vi "checkAlignment.vi"(5 "Ball":refnum<class "Ball.lvclass">, 6 "target gap":dbl[](array[numeric]), 7 "attacking ourselves":bool, 8 "error in (no error)":errorcluster, 9 "AlignError":T1, 10 "Robot":refnum<class "Robot.lvclass">, 11 "KickToSkill in":refnum<class "KickToSkill.lvclass">) -> (0 "error out":errorcluster, 2 "Aligned":bool, 3 "KickToSkill out":refnum<class "KickToSkill.lvclass">)   [LabVIEW 2023, in "KickToSkill.lvclass"]
uses:
  KickToSkill.lvclass
  Robot_class/Robot.lvclass
  Ball_class/Ball.lvclass
  Robot_class/robotKickToStates.ctl
  Robot_class/Robot.lvclass/Robot.ctl
  Object_class/Read position(x,y).vi
  Robot_class/Read robotKickState.vi
  Robot_class/Read orientation.vi
  Utilities_class/Utilities.lvclass
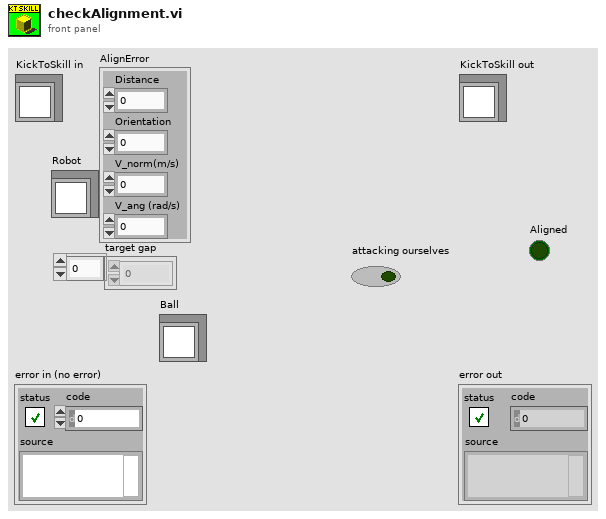
[diagram p1: front panel]
types:
  T1 = cluster{"Distance":dbl, "Orientation":dbl, "V_norm(m/s)":dbl, "V_ang (rad/s)":dbl}
  T2 = typedef "robotKickToStates.ctl" = enum16{"shootFromDirect", "avoidCollideBall", "goToBackBall", "none", "walk", "turn", "turnAntiClockWise", "turnClockwise", "oldKickToShoot", "oldKickToGoToBackBall", "shoot"}
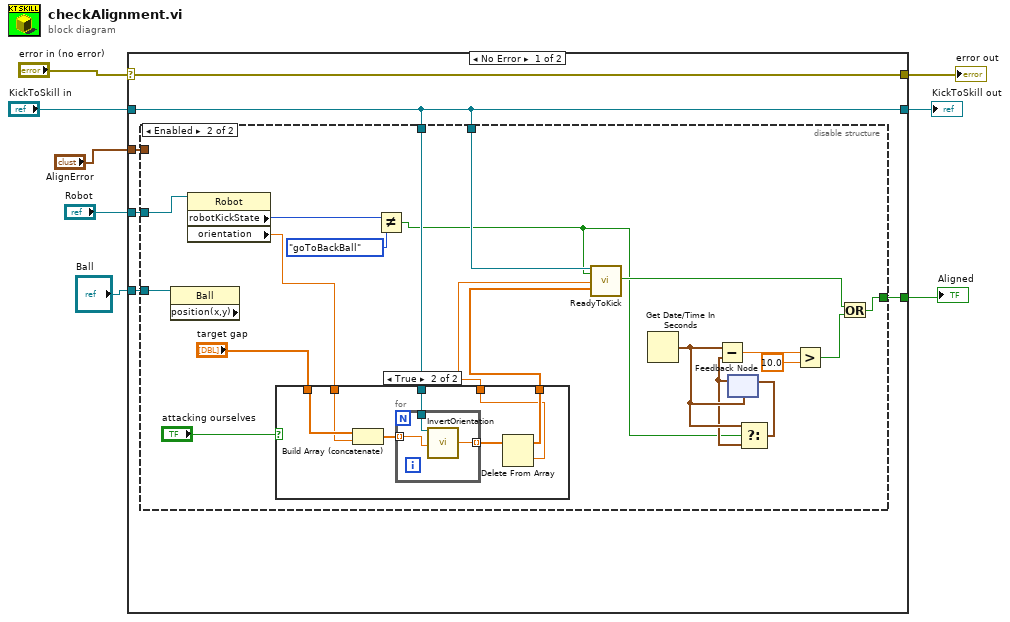
[diagram p0: block diagram]
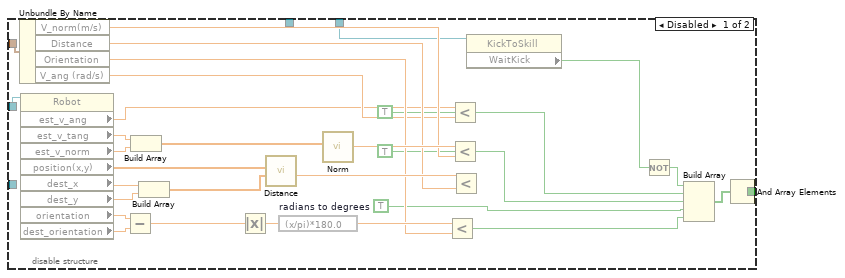
[diagram p2: hidden frame]
diagram:
  n1 = case shown="No Error" "error in (no error)" {
    selector: "error in (no error)" -> [w14 w78]
    tunnel: [w14 w78] -> w7
    tunnel: [w10 w77] -> w5
    tunnel: "KickToSkill in" -> [w10 w77]
    tunnel: "Robot" -> [w13 _]
    tunnel: "AlignError" -> [w12 _]
    tunnel: [w11 _] -> w2
    tunnel: "Ball" -> [w9 _]
    frame No Error {
      n2 = disable-structure shown="Enabled" {
        disable-tunnel: w13 -> [w44 w63]
        disable-tunnel: w12 -> [w29 _]
        disable-tunnel: w10 -> [w23 w64]
        disable-tunnel: [w18 w48] -> w11
        disable-tunnel: w10 -> [_ w57]
        disable-tunnel: w9 -> [_ w56]
        frame Disabled {
          n3 = Unbundle By Name(w29) -> ("V_norm(m/s)"=w28:dbl, "Distance"=w27:dbl, "Orientation"=w26:dbl, "V_ang (rad/s)"=w25:dbl)
          n4 = property class="Robot"(reference=w44) -> ("est_v_ang"=w24:dbl, "est_v_tang"=w32:dbl, "est_v_norm"=w33:dbl, "position(x,y)"=w40:dbl[], "dest_x"=w43:dbl, "dest_y"=w42:dbl, "orientation"=w39:dbl, "dest_orientation"=w38:dbl)  [unwired: 1 in, 2 out]
          n5 = Subtract(x=w39, y=w38) -> (x-y=w37:dbl)
          n6 = Build Array(w32, w33) -> (w31:dbl[])
          n7 = Build Array(w43, w42) -> (w41:dbl[])
          n8 = Absolute Value(x=w37) -> (abs(x)=w36:dbl)
          n9 = call "Distance.vi"("P1"=w41, "P2"=w40) -> ("Distance"=w34:dbl)  [unwired: 7 in, 2 out]
          n10 = expression code="(x/pi)*180.0" "radians to degrees"(w36) -> (w35:dbl)
          n11 = call "Norm.vi"("2D vector"=w31) -> ("Modulo"=w30:dbl)  [unwired: 8 in, 2 out]
          n12 = Less?(x=w35, y=w26) -> (x < y?=w20:bool)
          n13 = Less?(x=w24, y=w25) -> ()  [unwired: 1 out]
          n14 = Less?(x=w30, y=w28) -> ()  [unwired: 1 out]
          n15 = Less?(x=w34, y=w27) -> ()  [unwired: 1 out]
          n16 = property class="KickToSkill"(reference=w23) -> ("WaitKick"=w22:bool)  [unwired: 1 in, 2 out]
          n17 = Not(x=w22) -> (.not. x?=w21:bool)
          n18 = Build Array(w21, TRUE, TRUE, TRUE, w20) -> (w19:bool[])
          n19 = And Array Elements(Boolean array=w19) -> (logical AND=w18:bool)
        }
        frame Enabled {
          n20 = property class="Ball" props=["position(x,y)"](reference=w56) -> ()  [unwired: 1 in, 3 out]
          n21 = property class="Robot"(reference=w63) -> ("robotKickState"=w47:T2, "orientation"=w59:dbl)  [unwired: 1 in, 2 out]
          n22 = case shown="True" "attacking ourselves" {
            tunnel: [w66 w69] -> w60
            tunnel: "target gap" -> [w66 w73]
            tunnel: w59 -> [w65 w70]
            tunnel: [w65 w68] -> w58
            tunnel: w57 -> [_ w67]
            frame False {
            }
            frame True {
              n23 = Build Array (concatenate)(w73, w70) -> (w72:dbl[])
              n24 = for {
                tunnel: w72 -> [w76] mode=indexing
                tunnel: [w75] -> w71 mode=indexing
                tunnel: w67 -> [w74]
                n25 = call "InvertOrientation.vi"("object in"=w74, "orientation"=w76) -> ("inverted"=w75:dbl)  [unwired: 15 in, 2 out]
              }
              n26 = Delete From Array(array=w71) -> (deleted portion=w68:dbl, array with subset deleted=w69:dbl[])  [unwired: 2 in]
            }
          }
          n27 = Not Equal?(x=w47, y=robotKickToStates."goToBackBall") -> (x != y?=w45:bool)
          n28 = call "ReadyToKick.vi"("object in"=w64, "first call?"=w45, "dest_orientation"=w58, "target gap"=w60) -> ("kick"=w49:bool)  [unwired: 13 in, 2 out]
          n29 = Get Date/Time In Seconds() -> (seconds since 1Jan1904=w54:timestamp)
          n30 = feedback #1(w54) -> (w53:timestamp)
          n31 = Subtract(x=w54, y=w53) -> (x-y=w55:dbl)
          n32 = Select(t=w54, s=w45, f=w53) -> (s? t:f=w52:timestamp)
          n33 = feedback-in #1(w52) -> ()
          n34 = Greater?(x=w55, y=10.0) -> (0:w50:bool)
          n35 = Or(x=w49, y=w50) -> (x .or. y?=w48:bool)
        }
      }
    }
    frame Error {
    }
  }
  "error out" <- w7
  "KickToSkill out" <- w5
  "Aligned" <- w2
